vi "CloseBaxterCamera.vi"(3 "error in":errorcluster, 4 "Camera":T1, 5 "node":string) -> (0 "error out":errorcluster, 1 "Error Code":i32, 2 "OK?":bool)   [LabVIEW 2013]
uses:
  ROS/Code/SubVIs/BaxterCamera.ctl
  ROS/MessageBuilding/Primitives/subs/stringScalar.vi
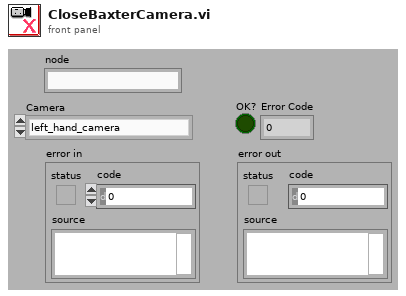
[diagram p1: front panel]
types:
  T1 = typedef "BaxterCamera.ctl" = enum16{"left_hand_camera", "right_hand_camera", "head_camera"}
  T2 = typedef "_ROSControl.ctl" = cluster{"topic port":u16, "Node":string, "topic":string, "type":string, "node port":u32, "error ":errorcluster, "Direction":T3, "APIs":string[]}
  T3 = typedef "_ROSDirection.ctl" = enum16{"Node", "Publisher", "Subscriber", "Service Client"}
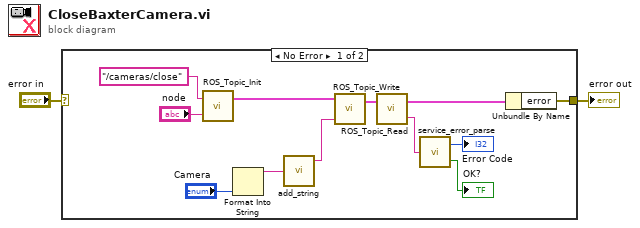
[diagram p0: block diagram]
diagram:
  n1 = case shown="No Error" "error in" {
    selector: "error in" -> [_ w15]
    tunnel: [w14 w15] -> w2
    frame No Error {
      n2 = call "ROS_Topic_Init.vi"("node"="node", "topic"="/cameras/close") -> ("ROS out"=w12:T2)  [unwired: 1 in]
      n3 = Format Into String("Camera") -> (resulting string=w3:string)  [unwired: 3 in, 1 out]
      n4 = call-poly "add_string.vi"("String"=w3) -> ("msg out"=w5:string)  [unwired: 4 in]
      n5 = call "ROS_Topic_Write.vi"("Msg in"=w5, "ROS in"=w12) -> ("ROS out"=w10:T2)  [unwired: 2 in]
      n6 = call "ROS_Topic_Read.vi"("ROS in"=w10) -> ("Reply"=w8:string, "ROS out"=w9:T2)  [unwired: 1 in]
      n7 = call "service_error_parse.vi"("Reply"=w8) -> ("OK?"=→"OK?":bool, "Error Code"=→"Error Code":i32)
      n8 = Unbundle By Name(w9) -> ("error"=w14:errorcluster)
    }
    frame Error {
    }
  }
  "error out" <- w2
